vi "Write Horizontal Settings.vi"(8 "error in (no error)":errorcluster, 10 "Horizontal Settings":T1={"Continuous"=FALSE, "EnableAveraging"=FALSE, "Number Averages"=0, "Measurement Timeout"=0.0, "Min Record Length"=1000, "Min Sample Rate"=10000000.0, "Enforce Realtime"=TRUE, "Sampling Mode "=enum."Real Time", "Interpolation"=enum."No Interpolation", "Type"=enum."Normal", "StartTime"=0.0, "Time Per Record"=0.0} {"Min Sample Rate" step=1000000.0 format="%#.2p"}, 11 "ScopePluginsBase in":refnum<class "ScopePluginsBase.lvclass">) -> (0 "error out":errorcluster, 3 "ScopePluginsBase out":refnum<class "ScopePluginsBase.lvclass">)   [LabVIEW 2018, in "ScopePlugins.lvlib" / "ScopePluginsBase.lvclass"]
uses:
  ScopePluginsBase.lvclass
  Typedefs/HorizontalSettings.ctl
  ScopePluginsBase.lvclass/ScopePluginsBase.ctl
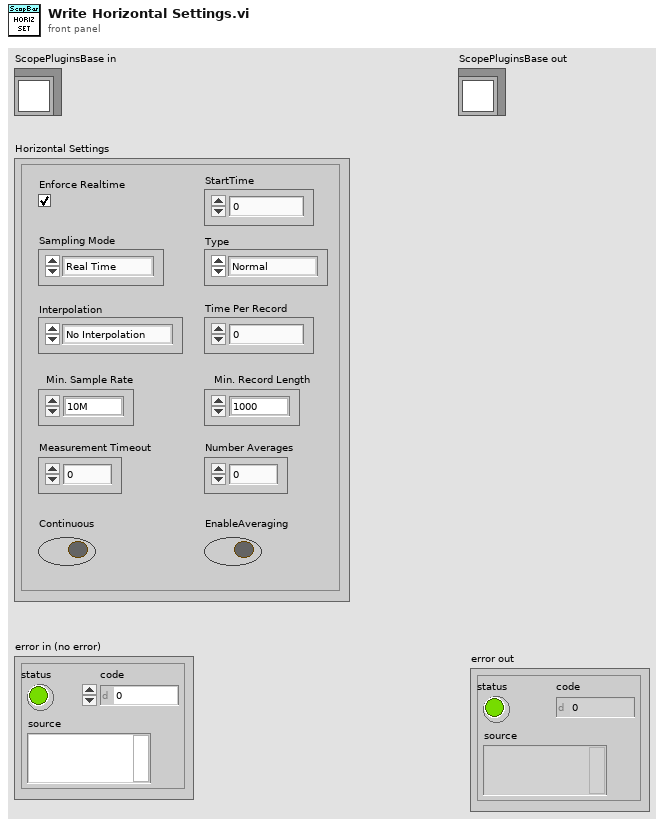
[diagram p1: front panel]
types:
  T1 = typedef "ScopePlugins.lvlib/ScopePluginsBase.lvclass/HorizontalSettings.ctl" = cluster{"Continuous":bool, "EnableAveraging":bool, "Number Averages":i32, "Measurement Timeout":dbl, "Min Record Length":i32, "Min Sample Rate":dbl, "Enforce Realtime":bool, "Sampling Mode ":enum16{"Real Time", "Equivalent Time", "Segment", "Real Time Peak Detect", "Real Time High Resolution", "Peak Detect Segment", "High Resolution Segment"}, "Interpolation":enum16{"No Interpolation", "sin(x)/x", "linear", "1 Point sin(x)/x", "2 Point sin(x)/x", "4 Point sin(x)/x", "8 Point sin(x)/x", "16 Point sin(x)/x"}, "Type":enum16{"Normal", "PeakDetect", "HighRes", "Envelope", "Average"}, "StartTime":dbl, "Time Per Record":dbl}
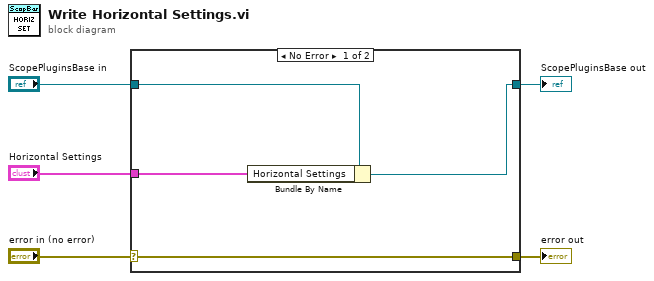
[diagram p0: block diagram]
diagram:
  n1 = case shown="No Error" "error in (no error)" {
    selector: "error in (no error)" -> [w9 w10]
    tunnel: [w9 w10] -> w4
    tunnel: [w7 w11] -> w2
    tunnel: "ScopePluginsBase in" -> [w8 w11]
    tunnel: "Horizontal Settings" -> [w6 _]
    frame No Error {
      n2 = Bundle By Name(cluster=w8, "Horizontal Settings"=w6) -> (w7:refnum<class "ScopePluginsBase.lvclass">)
    }
    frame Error {
    }
  }
  "error out" <- w4
  "ScopePluginsBase out" <- w2
